vi "InsertNode.vi"(6 "k":i32=1, 7 "Algorithm":enum16{"RRT", "A*"}(ring), 8 "Depth":i32=1, 10 "New Node":dbl[](array[numeric]), 11 "Tree":dbl[][](array[numeric])) -> (2 "New Tree":dbl[][](array[numeric]))   [LabVIEW 2016]
uses:
  Node.ctl
panel:
  in  "index":i32
  in  "Node":T1
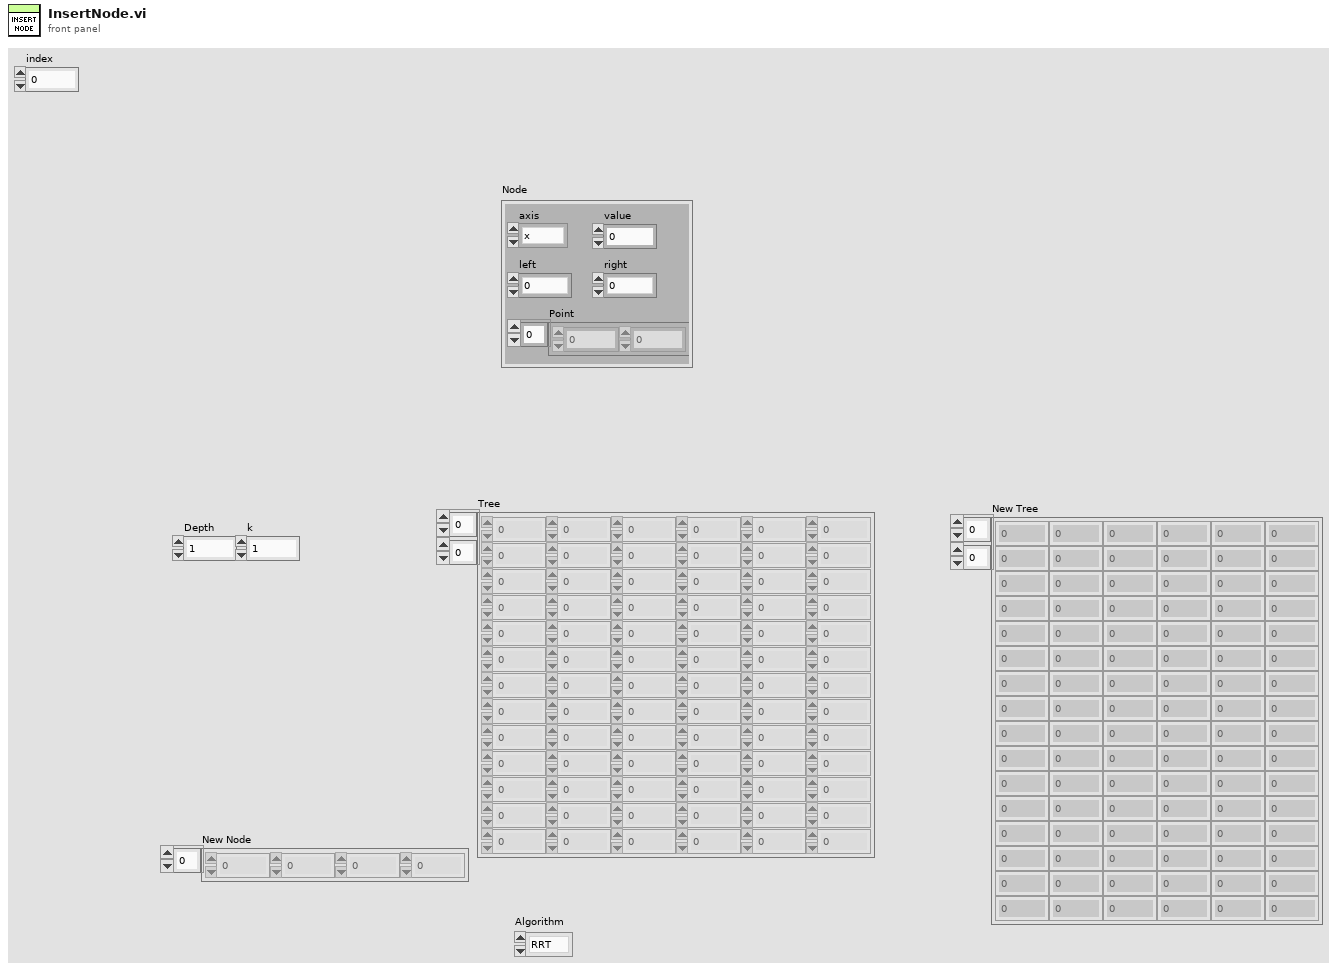
[diagram p1: front panel]
types:
  T1 = typedef "Node.ctl" = cluster{"axis":enum16{"x", "y"}, "value":dbl, "left":dbl, "right":dbl, "Point":dbl[]}
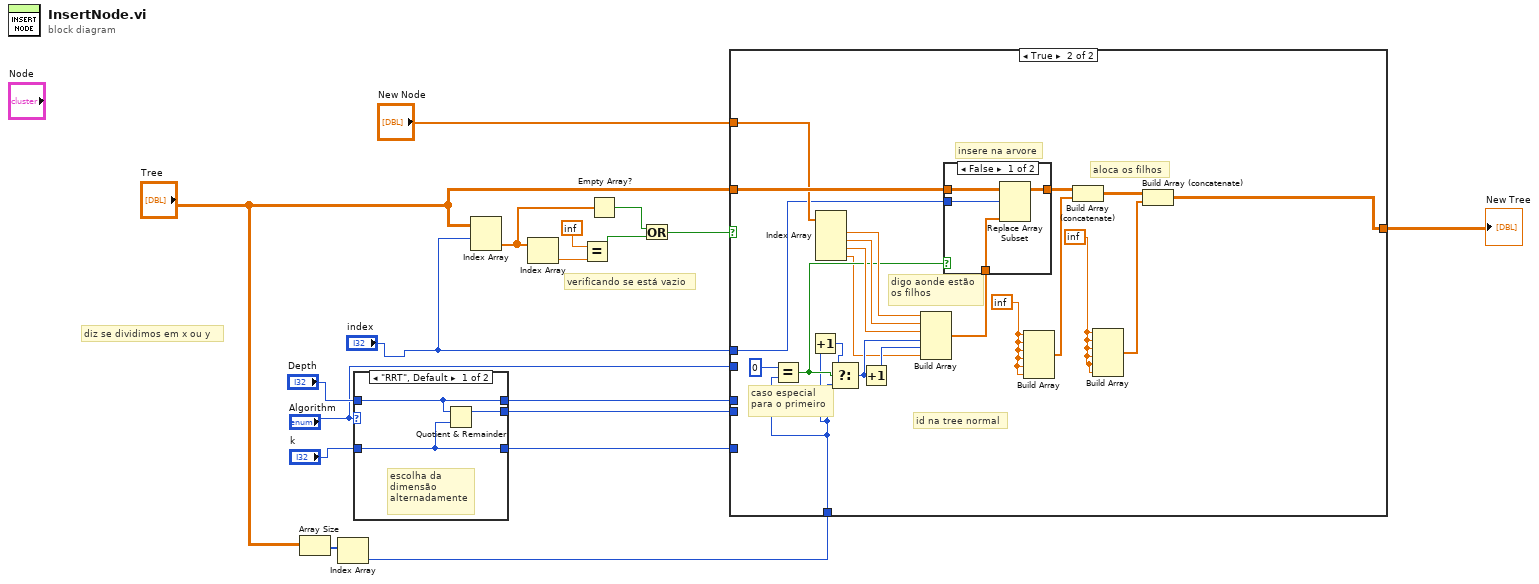
[diagram p0: block diagram]
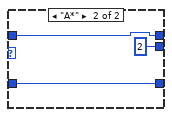
[diagram p2: hidden frame]
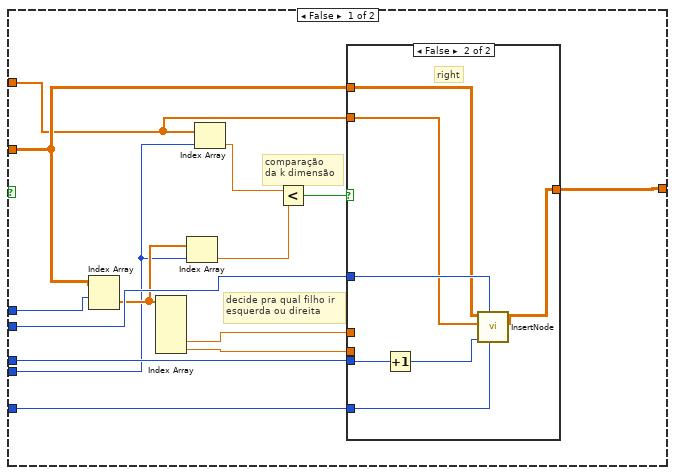
[diagram p3: hidden frame]
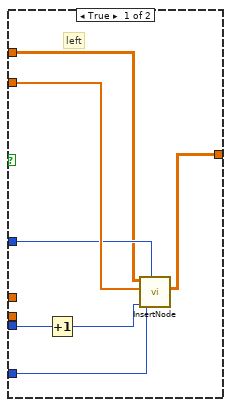
[diagram p4: hidden frame]
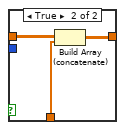
[diagram p5: hidden frame]
diagram:
  # "diz se dividimos em x ou y"
  # "verificando se está vazio"
  n1 = Array Size(array="Tree") -> (size(s)=w8:i32[])
  n2 = Index Array(array=w8) -> (element=w2:i32)  [unwired: 1 in]
  n3 = case shown="\"RRT\", Default" "Algorithm" {
    tunnel: [w21 2] -> w18
    tunnel: [w20 w22] -> w17
    tunnel: [w19 w24] -> w15
    tunnel: "Depth" -> [w20 w22]
    tunnel: "k" -> [w19 w24]
    frame "RRT", Default {
      # "escolha da \ndimensão \nalternadamente"
      n4 = Quotient & Remainder(x=w20, y=w19) -> (x-y*floor(x/y)=w21:i32)  [unwired: 1 out]
    }
    frame "A*" {
    }
  }
  n5 = Index Array(array="Tree", index (row)="index") -> (element=w7:dbl[])  [unwired: 1 in]
  n6 = Index Array(array=w7) -> (element=w13:dbl)  [unwired: 1 in]
  n7 = Equal?(x=inf, y=w13) -> (x = y?=w5:bool)
  n8 = Empty Array?(array=w7) -> (empty?=w6:bool)
  n9 = Or(x=w6, y=w5) -> (x .or. y?=w4:bool)
  n10 = case shown="True" w4 {
    tunnel: w18 -> [w26 _]
    tunnel: "Tree" -> [w36 w73]
    tunnel: "index" -> [w35 w67]
    tunnel: w17 -> [w34 _]
    tunnel: "New Node" -> [w33 w69]
    tunnel: w15 -> [w32 _]
    tunnel: [w31 w61] -> w12
    tunnel: "Algorithm" -> [w28 _]
    tunnel: w2 -> [_ w57]
    frame False {
      # "decide pra qual filho ir\nesquerda ou direita"
      # "comparação\nda k dimensão"
      n11 = Index Array(array=w36, index (row)=w35) -> (element=w27:dbl[])  [unwired: 1 in]
      n12 = Index Array(array=w27) -> (element #4=w30:dbl, element #5=w29:dbl)  [unwired: 5 in, 3 out]
      n13 = Index Array(array=w27, index=w26) -> (element=w25:dbl)
      n14 = Index Array(array=w33, index=w26) -> (element=w38:dbl)
      n15 = Less?(x=w38, y=w25) -> (x < y?=w37:bool)
      n16 = case shown="False" w37 {
        tunnel: w36 -> [w39 w47]
        tunnel: w34 -> [w45 w52]
        tunnel: w33 -> [w43 w46]
        tunnel: w32 -> [w42 w50]
        tunnel: [w41 w49] -> w31
        tunnel: w30 -> [_ _]
        tunnel: w29 -> [_ _]
        tunnel: w28 -> [w40 w48]
        frame True {
          # "left"
          n17 = Increment(x=w45) -> (x+1=w44:i32)
          n18 = call "InsertNode.vi"("k"=w42, "Algorithm"=w40, "Depth"=w44, "New Node"=w43, "Tree"=w39) -> ("New Tree"=w41:dbl[][])  [unwired: 6 in]
        }
        frame False {
          # "right"
          n19 = Increment(x=w52) -> (x+1=w51:i32)
          n20 = call "InsertNode.vi"("k"=w50, "Algorithm"=w48, "Depth"=w51, "New Node"=w46, "Tree"=w47) -> ("New Tree"=w49:dbl[][])  [unwired: 6 in]
        }
      }
    }
    frame True {
      w54 = inf
      w53 = inf
      # "id na tree normal"
      # "digo aonde estão\nos filhos"
      # "caso especial\npara o primeiro"
      # "insere na arvore"
      # "aloca os filhos"
      n21 = Equal?(x=0, y=w57) -> (x = y?=w59:bool)
      n22 = Increment(x=w57) -> (x+1=w56:i32)
      n23 = Index Array(array=w69) -> (element #1=w72:dbl, element #2=w71:dbl, element #3=w70:dbl, element #4=w55:dbl)  [unwired: 4 in]
      n24 = Select(t=w56, s=w59, f=w57) -> (s? t:f=w58:i32)
      n25 = Increment(x=w58) -> (x+1=w66:i32)
      n26 = Build Array(w72, w71, w70, w58, w66, w55) -> (w68:dbl[])
      n27 = case shown="False" w59 {
        tunnel: w73 -> [w77 w80]
        tunnel: w68 -> [w76 w79]
        tunnel: w67 -> [w75 _]
        tunnel: [w74 w78] -> w65
        frame False {
          n28 = Replace Array Subset(array=w77, new element=w76, index (row)=w75) -> (w74:dbl[][])  [unwired: 1 in]
        }
        frame True {
          n29 = Build Array (concatenate)(w80, w79) -> (w78:dbl[][])
        }
      }
      n30 = Build Array(w54, w54, w54, w54, w54, w54) -> (w64:dbl[])
      n31 = Build Array (concatenate)(w65, w64) -> (w63:dbl[][])
      n32 = Build Array(w53, w53, w53, w53, w53, w53) -> (w62:dbl[])
      n33 = Build Array (concatenate)(w63, w62) -> (w61:dbl[][])
    }
  }
  "New Tree" <- w12
